vi "XML - Evaluate Rx Imported Channels.vi"(8 "error in (no error)":errorcluster, 10 "Channel Info Array":T1[](array[typedef]) {"Data Type" items=["U8", "U16", "U32", "U64", "I8", "I16", "I32", "I64", "SGL", "DBL", "EXT"]}, 11 "Node Ptr in":u64 format="%.0x") -> (0 "error out":errorcluster, 2 "Invalid Channels":string[](array[string]), 3 "Node Ptr out":u64 format="%.0x")   [LabVIEW 2016, in "UDP-Custom-Device System Explorer.lvlib"]
uses:
  UDP-Custom-Device System Explorer.lvlib
  Types/XML/XML - Channel.ctl
  <vilib>/NI Veristand/Custom Device API/Custom Device Item Ref.ctl
  Shared/Constants.vi
  <vilib>/NI Veristand/Custom Device Tools/Custom Device Utility Library/NI VeriStand - Search for Item by GUID.vi
  <vilib>/NI VeriStand/Custom Device Tools/Custom Device Utility Library/Custom Device Utility Library.lvlib
  <vilib>/NI VeriStand/Custom Device API/Custom Device API.lvlib
  Shared/UDP-Custom-Device Shared.lvlib
  Property Accessors/Shared Packet Accessors.lvlib
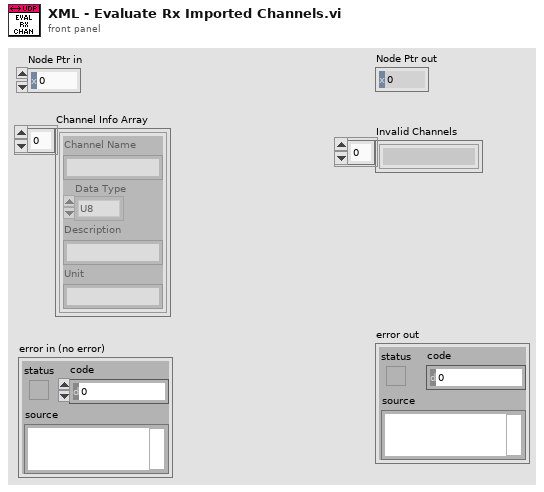
[diagram p1: front panel]
types:
  T1 = typedef "UDP-Custom-Device System Explorer.lvlib/XML - Channel.ctl" = cluster{"Channel Name":string, "Data Type":u16, "Description":string, "Unit":string}
  T2 = typedef "Custom Device API.lvlib/Custom Device Item Ref.ctl" = u64
  T3 = cluster{"Channel Names":string[], "Channel Paths":string[], "Dependent Node References":T2[]}
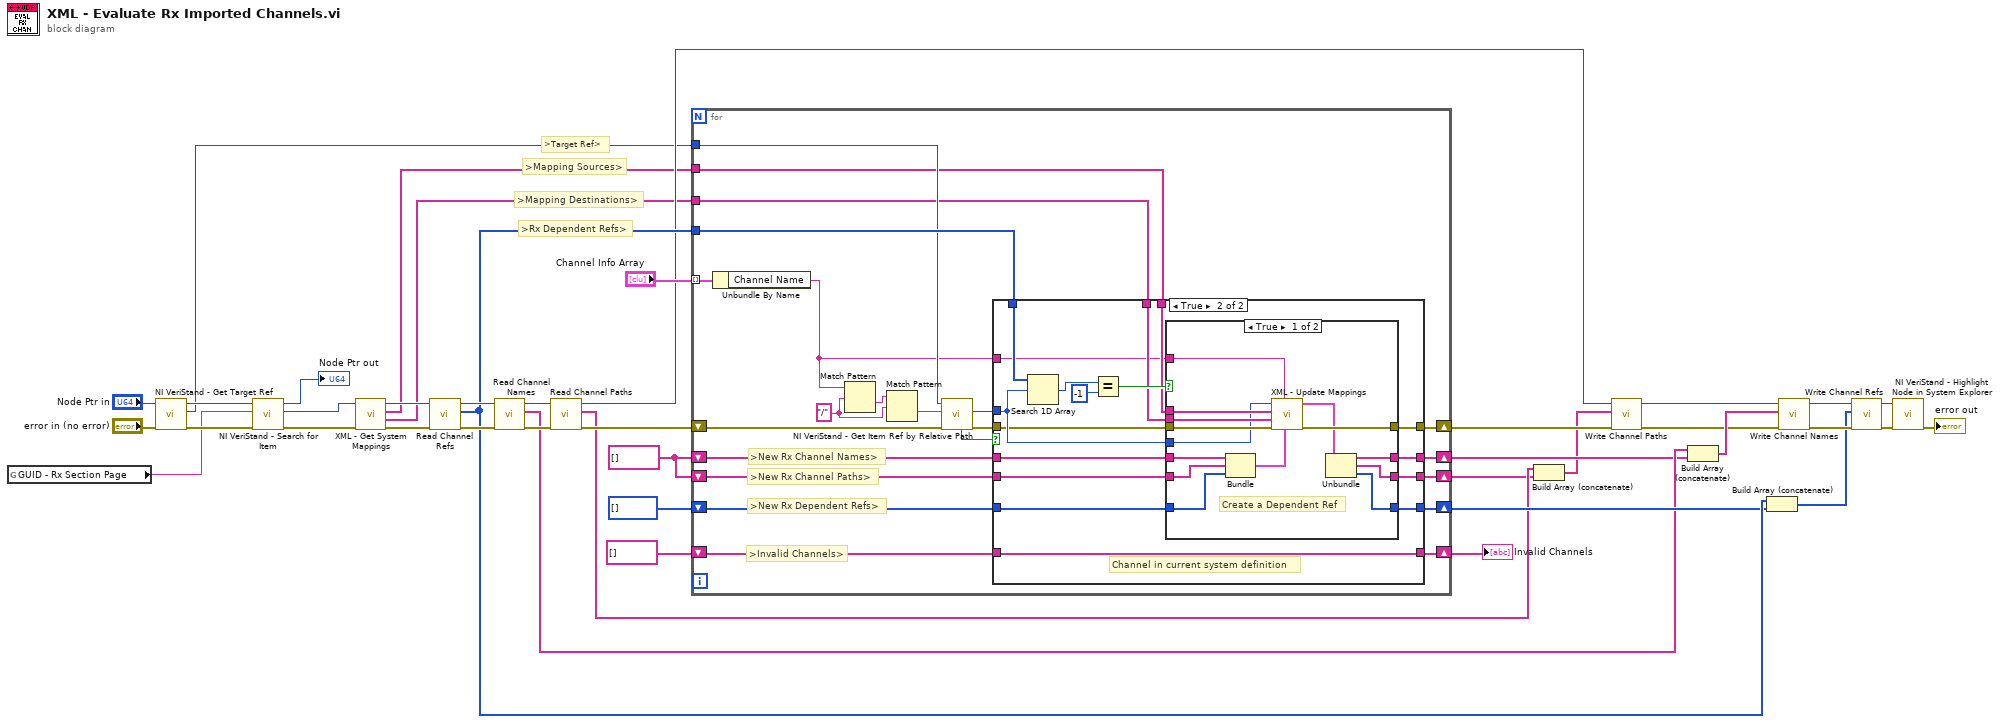
[diagram p0: block diagram]
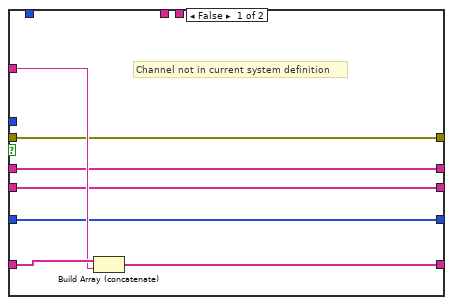
[diagram p2: hidden frame]
diagram:
  w31 = string[] []
  # ">Rx Dependent Refs>"
  # ">Mapping Destinations>"
  # ">Mapping Sources>"
  # ">Target Ref>"
  n1 = global read "Constants.vi" "GUID - Rx Section Page"() -> (w1:string)
  n2 = call <vilib>:"NI VeriStand - Get Target Ref.vi"("error in"="error in (no error)", "Item Ref in"="Node Ptr in") -> ("error out"=w11:errorcluster, "Target Ref"=w8:T2, "Item Ref out"=w9:T2)  [unwired: 6 in, 1 out]
  n3 = call-poly <vilib>:"NI VeriStand - Search for Item.vi"("error in"=w11, "Item GUID"=w1, "Section Ref in"=w9) -> ("error out"=w6:errorcluster, "Item Ref"=w7:T2, "Section Ref out"=→"Node Ptr out":T2)  [unwired: 5 in, 1 out]
  n4 = call "XML - Get System Mappings.vi"("error in (no error)"=w6, "Item Ref in"=w7) -> ("error out"=w5:errorcluster, "Channel Path Destinations"=w3:string[], "Channel Path Sources"=w2:string[], "Item Ref out"=w4:T2)  [unwired: 6 in]
  n5 = call "Read Channel Refs.vi"("error in (no error)"=w5, "Node Ptr"=w4) -> ("error out"=w37:errorcluster, "Dependent Node Refs"=w30:T2[], "Node Ptr out"=w36:T2)  [unwired: 7 in]
  n6 = call "Read Channel Names.vi"("error in (no error)"=w37, "Node Ptr"=w36) -> ("error out"=w35:errorcluster, "Channel Names"=w28:string[], "Node Ptr out"=w34:T2)  [unwired: 7 in]
  n7 = call "Read Channel Paths.vi"("error in (no error)"=w35, "Node Ptr"=w34) -> ("error out"=w33:errorcluster, "Channel Paths"=w26:string[], "Node Ptr out"=w23:T2)  [unwired: 7 in]
  n8 = for {
    tunnel: "Channel Info Array" -> [w63] mode=indexing
    shift-right: [w62] -> w24
    shift-left: w33 -> [w52]
    shift-right: [w60] -> w39
    shift-left: string[] [] -> [w61]
    tunnel: w30 -> [w59]
    shift-right: [w57] -> w29
    shift-left: T2[] [] -> [w58]
    shift-right: [w55] -> w27
    shift-left: w31 -> [w56]
    shift-right: [w53] -> w25
    shift-left: w31 -> [w54]
    tunnel: w8 -> [w50]
    tunnel: w3 -> [w43]
    tunnel: w2 -> [w42]
    w45 = "/" ("regular expression")
    # ">Invalid Channels>"
    # ">New Rx Channel Names>"
    # ">New Rx Channel Paths>"
    # ">New Rx Dependent Refs>"
    n9 = Unbundle By Name(w63) -> ("Channel Name"=w47:string)
    n10 = Match Pattern(string=w47, regular expression=w45) -> (after substring=w46:string)  [unwired: 1 in, 3 out]
    n11 = Match Pattern(string=w46, regular expression=w45) -> (after substring=w44:string)  [unwired: 1 in, 3 out]
    n12 = call <vilib>:"NI VeriStand - Get Item Ref by Relative Path.vi"("error in"=w52, "Relative Item Path"=w44, "Section Ref in"=w50) -> ("error out"=w51:errorcluster, "Item Ref"=w49:T2, "Found"=w48:bool)  [unwired: 5 in, 1 out]
    n13 = case shown="True" w48 {
      tunnel: w51 -> [w67 w79]
      tunnel: [w67 w74] -> w62
      tunnel: w61 -> [w70 w87]
      tunnel: w47 -> [w69 w71]
      tunnel: [w68 w87] -> w60
      tunnel: w59 -> [_ w86]
      tunnel: w49 -> [_ w81]
      tunnel: w58 -> [w66 w82]
      tunnel: [w66 w80] -> w57
      tunnel: w56 -> [w65 w78]
      tunnel: [w65 w77] -> w55
      tunnel: w54 -> [w64 w76]
      tunnel: [w64 w75] -> w53
      tunnel: w43 -> [_ w73]
      tunnel: w42 -> [_ w72]
      frame False {
        # "Channel not in current system definition"
        n14 = Build Array (concatenate)(w70, w69) -> (w68:string[])
      }
      frame True {
        # "Channel in current system definition"
        n15 = Search 1D Array(1D array=w86, element=w81) -> (index of element=w85:i32)  [unwired: 1 in]
        n16 = Equal?(x=w85, y=-1) -> (x = y?=w83:bool)
        n17 = case shown="True" w83 {
          tunnel: w82 -> [w98 w104]
          tunnel: w81 -> [w88 _]
          tunnel: [w91 w104] -> w80
          tunnel: w79 -> [w101 w105]
          tunnel: w78 -> [w100 w103]
          tunnel: [w93 w103] -> w77
          tunnel: w76 -> [w99 w102]
          tunnel: [w92 w102] -> w75
          tunnel: [w95 w105] -> w74
          tunnel: w73 -> [w96 _]
          tunnel: w72 -> [w97 _]
          tunnel: w71 -> [w89 _]
          frame True {
            # "Create a Dependent Ref"
            n18 = Bundle(w100, w99, w98) -> (w90:cluster{string[], string[], T2[]})  [unwired: 1 in]
            n19 = call "XML - Update Mappings.vi"("Channel Data in"=w90, "Channel Path"=w89, "error in (no error)"=w101, "Channel Path Destinations"=w96, "Channel Path Sources"=w97, "Item Ref in"=w88) -> ("error out"=w95:errorcluster, "Channel Data out"=w94:T3)  [unwired: 4 in]
            n20 = Unbundle(w94) -> ("Channel Names"=w93:string[], "Channel Paths"=w92:string[], "Dependent Node References"=w91:T2[])
          }
          frame False {
            # "Channel is a Dependent Ref"
          }
        }
      }
    }
  }
  "Invalid Channels" <- w39
  n21 = Build Array (concatenate)(w26, w25) -> (w22:string[])
  n22 = call "Write Channel Paths.vi"("error in (no error)"=w24, "Channel Paths"=w22, "Node Ptr"=w23) -> ("error out"=w19:errorcluster, "Node Ptr out"=w21:T2)  [unwired: 7 in]
  n23 = Build Array (concatenate)(w28, w27) -> (w20:string[])
  n24 = Build Array (concatenate)(w30, w29) -> (w16:T2[])
  n25 = call "Write Channel Names.vi"("error in (no error)"=w19, "Channel Names"=w20, "Node Ptr"=w21) -> ("error out"=w18:errorcluster, "Node Ptr out"=w17:T2)  [unwired: 7 in]
  n26 = call "Write Channel Refs.vi"("error in (no error)"=w18, "Dependent Node Refs"=w16, "Node Ptr"=w17) -> ("error out"=w15:errorcluster, "Node Ptr out"=w14:T2)  [unwired: 7 in]
  n27 = call <vilib>:"NI VeriStand - Highlight Node in System Explorer.vi"("error in (no error)"=w15, "Item Ref in"=w14) -> ("error out"=→"error out":errorcluster)  [unwired: 8 in, 1 out]
